vi "Formatacao de Waveform.vi"(1 "Data in":T1={"Closed Loop Enabled"=FALSE, "Proportional valve 1"=0.0, "Proportional valve 2"=0.0, "Plant Control Variables"={"Tank 1 Level"=0.0, "Tank 2 Level"=0.0, "Tank 3 Level"=0.0, "Tank 4 Level"=0.0, "Pump 1"=0.0, "Pump 2"=0.0}, "Setpoints"={"Setpoint tank 1"=0.0, "Setpoint tank 2"=0.0}, "Controller"={"Control Algorithm selector"=enum."LQG-LTR", "K"={"A"=[[-4.94989, 0.0218181, -352.966, 23.8192, -3.10685, -0.000952287], [-0.0218181, -4.904857, 23.4819, -343.472, 0.000977323, -3.58066], [0.0389045, 0.0, -31.6573, 0.0287797, 0.0245405, 0.0], [0.0, 0.0381972, 0.0287797, -31.6573, 0.0, 0.0280468], [0.0, 0.0325383, 0.0240248, -0.0293675, -0.0245405, 0.0], [0.031831, 0.0, -0.0282058, 0.0, 0.0, 0.0]], "B"=[[28.0692, -23.9099], [-23.3912, 28.5852], [31.6468, -0.0287797], [-0.0287797, 31.6468], [-0.0282058, -0.0293675], [0.0282058, -0.0240214]], "C"=[[4.94989, 0.0218181, 314.896, 0.0907351, 3.10685, 0.000952287], [10.0218181, 4.90457, -0.0906726, 314.884, -0.000977323, 3.58066]], "D"=[[0.0, 0.0], [0.0, 0.0]]}, "PI/W1"={"A"=[[-4.94989, 0.0218181, -352.966, 23.8192, -3.10685, -0.000952287], [-0.0218181, -4.904857, 23.4819, -343.472, 0.000977323, -3.58066], [0.0389045, 0.0, -31.6573, 0.0287797, 0.0245405, 0.0], [0.0, 0.0381972, 0.0287797, -31.6573, 0.0, 0.0280468], [0.0, 0.0325383, 0.0240248, -0.0293675, -0.0245405, 0.0], [0.031831, 0.0, -0.0282058, 0.0, 0.0, 0.0]], "B"=[[28.0692, -23.9099], [-23.3912, 28.5852], [31.6468, -0.0287797], [-0.0287797, 31.6468], [-0.0282058, -0.0293675], [0.0282058, -0.0240214]], "C"=[[4.94989, 0.0218181, 314.896, 0.0907351, 3.10685, 0.000952287], [10.0218181, 4.90457, -0.0906726, 314.884, -0.000977323, 3.58066]], "D"=[[0.0, 0.0], [0.0, 0.0]]}, "W2"={"A"=[[-4.94989, 0.0218181, -352.966, 23.8192, -3.10685, -0.000952287], [-0.0218181, -4.904857, 23.4819, -343.472, 0.000977323, -3.58066], [0.0389045, 0.0, -31.6573, 0.0287797, 0.0245405, 0.0], [0.0, 0.0381972, 0.0287797, -31.6573, 0.0, 0.0280468], [0.0, 0.0325383, 0.0240248, -0.0293675, -0.0245405, 0.0], [0.031831, 0.0, -0.0282058, 0.0, 0.0, 0.0]], "B"=[[28.0692, -23.9099], [-23.3912, 28.5852], [31.6468, -0.0287797], [-0.0287797, 31.6468], [-0.0282058, -0.0293675], [0.0282058, -0.0240214]], "C"=[[4.94989, 0.0218181, 314.896, 0.0907351, 3.10685, 0.000952287], [10.0218181, 4.90457, -0.0906726, 314.884, -0.000977323, 3.58066]], "D"=[[0.0, 0.0], [0.0, 0.0]]}}}) -> (0 "Tank Levels":waveform(dbl)[](array[waveform]))   [LabVIEW 2018]
uses:
  Real-Time/controls/Controller Data.ctl
  Real-Time/Control Algorithm/Control Algorithm Data.ctl
  Real-Time/Control Algorithm/Control Algorithm Selection.ctl
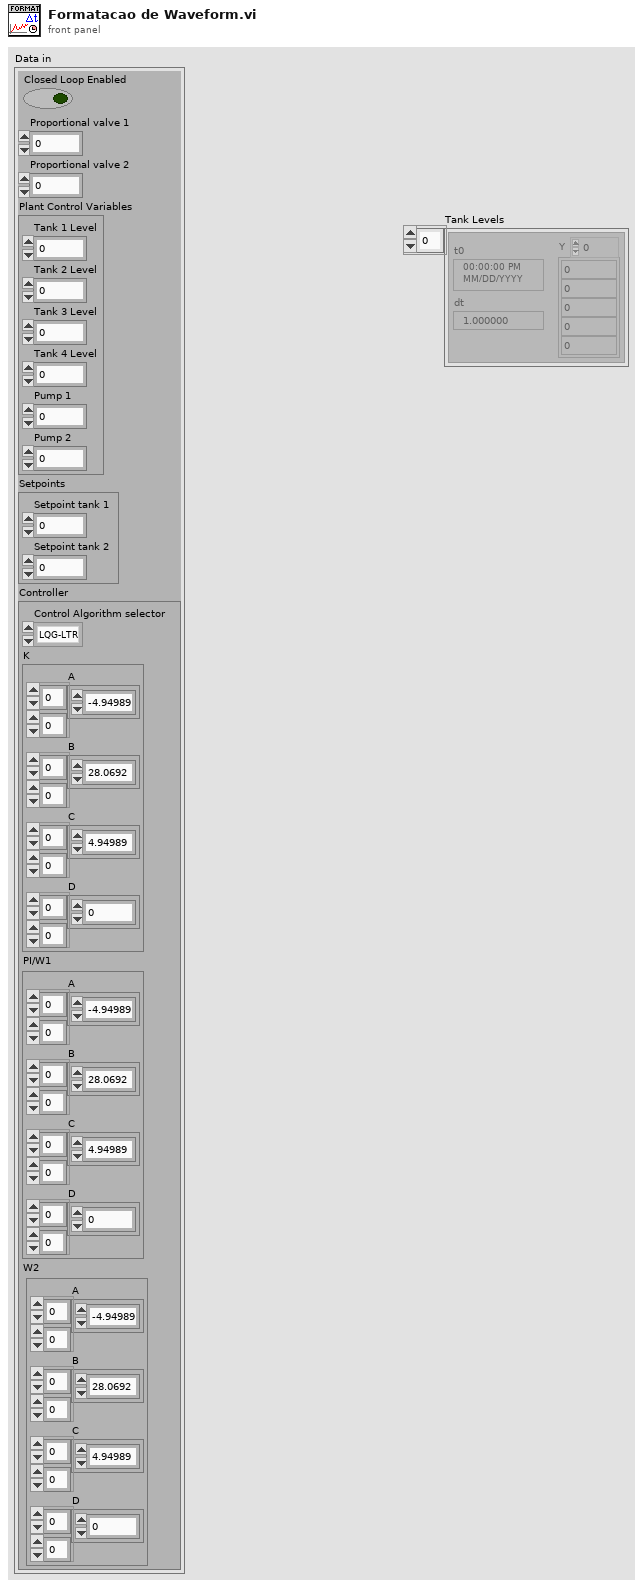
[diagram p1: front panel]
types:
  T1 = typedef "Controller Data.ctl" = cluster{"Closed Loop Enabled":bool, "Proportional valve 1":dbl, "Proportional valve 2":dbl, "Plant Control Variables":cluster{"Tank 1 Level":dbl, "Tank 2 Level":dbl, "Tank 3 Level":dbl, "Tank 4 Level":dbl, "Pump 1":dbl, "Pump 2":dbl}, "Setpoints":cluster{"Setpoint tank 1":dbl, "Setpoint tank 2":dbl}, "Controller":T2}
  T2 = typedef "Control Algorithm Data.ctl" = cluster{"Control Algorithm selector":T3, "K":cluster{"A":dbl[][], "B":dbl[][], "C":dbl[][], "D":dbl[][]}, "PI/W1":cluster{"A":dbl[][], "B":dbl[][], "C":dbl[][], "D":dbl[][]}, "W2":cluster{"A":dbl[][], "B":dbl[][], "C":dbl[][], "D":dbl[][]}}
  T3 = typedef "Control Algorithm Selection.ctl" = enum16{"LQG-LTR", "Hinf"}
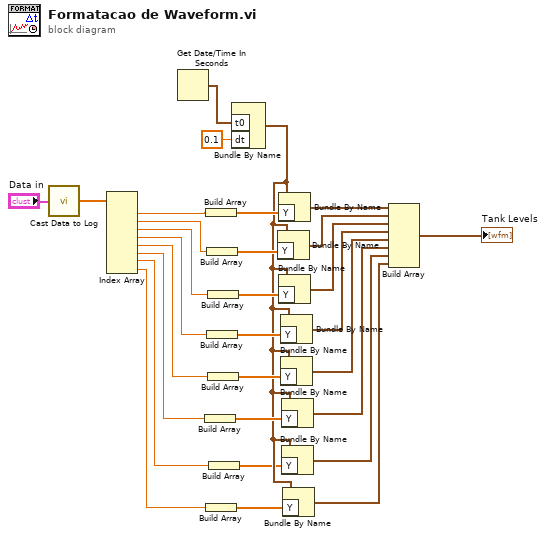
[diagram p0: block diagram]
diagram:
  n1 = call "Cast Data to Log.vi"("Data in"="Data in") -> ("Data out"=w2:dbl[])  [unwired: 4 in]
  n2 = Index Array(array=w2) -> (element #1=w26:dbl, element #2=w24:dbl, element #3=w23:dbl, element #4=w21:dbl, element #5=w19:dbl, element #6=w17:dbl, element #7=w6:dbl, element #8=w5:dbl)  [unwired: 8 in]
  n3 = Get Date/Time In Seconds() -> (seconds since 1Jan1904=w29:timestamp)
  n4 = Build Array(w17) -> (w16:dbl[])
  n5 = Build Array(w26) -> (w27:dbl[])
  n6 = Build Array(w5) -> (w9:dbl[])
  n7 = Build Array(w24) -> (w25:dbl[])
  n8 = Build Array(w21) -> (w20:dbl[])
  n9 = Build Array(w23) -> (w22:dbl[])
  n10 = Build Array(w19) -> (w18:dbl[])
  n11 = Build Array(w6) -> (w7:dbl[])
  n12 = Bundle By Name("t0"=w29, "dt"=0.1) -> (w8:waveform(dbl))  [unwired: 1 in]
  n13 = Bundle By Name(cluster=w8, "Y"=w25) -> (w10:waveform(dbl))
  n14 = Bundle By Name(cluster=w8, "Y"=w27) -> (w11:waveform(dbl))
  n15 = Bundle By Name(cluster=w8, "Y"=w22) -> (w30:waveform(dbl))
  n16 = Bundle By Name(cluster=w8, "Y"=w20) -> (w28:waveform(dbl))
  n17 = Bundle By Name(cluster=w8, "Y"=w18) -> (w15:waveform(dbl))
  n18 = Bundle By Name(cluster=w8, "Y"=w16) -> (w14:waveform(dbl))
  n19 = Bundle By Name(cluster=w8, "Y"=w7) -> (w4:waveform(dbl))
  n20 = Bundle By Name(cluster=w8, "Y"=w9) -> (w3:waveform(dbl))
  n21 = Build Array(w11, w10, w30, w28, w15, w14, w4, w3) -> (→"Tank Levels":waveform(dbl)[])
